vi "Pause Counter.vi"(8 "error in (no error)":errorcluster, 10 "ligne index":i32, 11 "Hardware Resources in":T1={"AI"={"task name"="", "task_ref"="", "physical channels"="Dev1/ai0:7", "channels config"={"input terminal configuration"=0, "minimum value"=-5.0, "maximum value"=5.0}, "rate"=1000.0}, "conversions"={"ai0"={"a"=0.0, "b"=0.0}, "ai1"={"a"=0.0, "b"=0.0}, "ai2"={"a"=0.0, "b"=0.0}, "ai3"={"a"=0.0, "b"=0.0}, "ai4"={"a"=0.0, "b"=0.0}}, "compteur 0"={"task name"="CTR", "task_ref"="", "ctr"="Dev1/ctr0:3", "coeff"=4000.0}, "compteur 1"={"task name"="CTR1", "task_ref"="", "ctr"="Dev1/ctr1", "coeff"=4000.0}, "compteur 2"={"task name"="CTR2", "task_ref"="", "ctr"="Dev1/ctr2", "coeff"=4000.0}, "compteur 3"={"task name"="CTR3", "task_ref"="", "ctr"="Dev1/ctr3", "coeff"=4000.0}} {"compteur 3"."coeff" format="%0.2f"; "compteur 2"."coeff" format="%0.2f"; "compteur 1"."coeff" format="%0.2f"; "compteur 0"."coeff" format="%0.2f"; "AI"."rate" format="%0.2f"; "AI"."channels config"."input terminal configuration" items=["Default"=-1, "RSE"=10083, "NRSE"=10078, "Differential"=10106, "Pseudodifferential"=12529]}) -> (0 "error out":errorcluster, 3 "Hardware Resources out":T1={"AI"={"task name"="", "task_ref"="", "physical channels"="Dev1/ai0:7", "channels config"={"input terminal configuration"=0, "minimum value"=-5.0, "maximum value"=5.0}, "rate"=1000.0}, "conversions"={"ai0"={"a"=0.0, "b"=0.0}, "ai1"={"a"=0.0, "b"=0.0}, "ai2"={"a"=0.0, "b"=0.0}, "ai3"={"a"=0.0, "b"=0.0}, "ai4"={"a"=0.0, "b"=0.0}}, "compteur 0"={"task name"="CTR", "task_ref"="", "ctr"="Dev1/ctr0:3", "coeff"=4000.0}, "compteur 1"={"task name"="CTR1", "task_ref"="", "ctr"="Dev1/ctr1", "coeff"=4000.0}, "compteur 2"={"task name"="CTR2", "task_ref"="", "ctr"="Dev1/ctr2", "coeff"=4000.0}, "compteur 3"={"task name"="CTR3", "task_ref"="", "ctr"="Dev1/ctr3", "coeff"=4000.0}} {"compteur 3"."coeff" format="%0.2f"; "compteur 2"."coeff" format="%0.2f"; "compteur 1"."coeff" format="%0.2f"; "compteur 0"."coeff" format="%0.2f"; "AI"."rate" format="%0.2f"; "AI"."channels config"."input terminal configuration" items=["Default"=-1, "RSE"=10083, "NRSE"=10078, "Differential"=10106, "Pseudodifferential"=12529]})   [LabVIEW 2014, in "PLS Acquisition.lvlib"]
doc: "Stops the acquisition."
uses:
  PLS Acquisition.lvlib
  Hardware Configuration.ctl
  Settings/conversion.ctl
  Settings/PLS Settings.lvlib
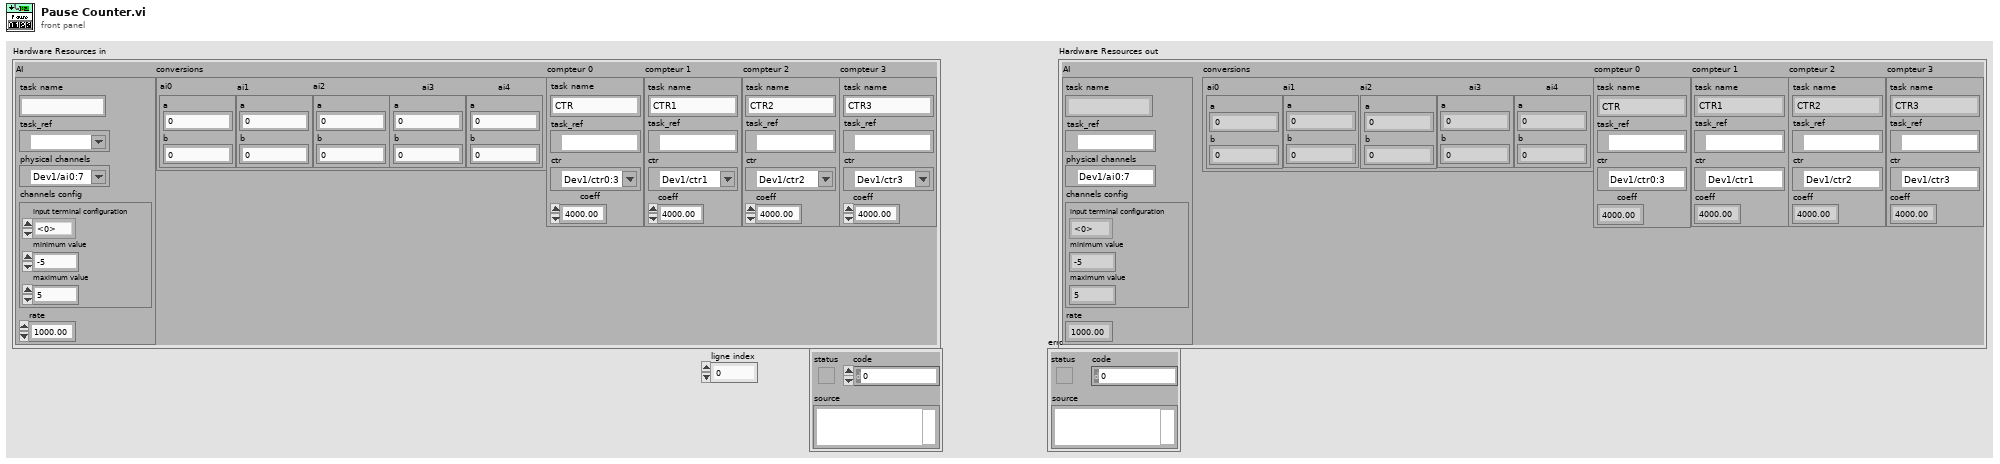
[diagram p1: front panel]
types:
  T1 = typedef "PLS Acquisition.lvlib/Hardware Configuration.ctl" = cluster{"AI":cluster{"task name":string, "task_ref":refnum<k21>, "physical channels":tag, "channels config":cluster{"input terminal configuration":i32, "minimum value":dbl, "maximum value":dbl}, "rate":dbl}, "conversions":cluster{"ai0":T2, "ai1":T2, "ai2":T2, "ai3":T2, "ai4":T2}, "compteur 0":cluster{"task name":string, "task_ref":refnum<k21>, "ctr":tag, "coeff":dbl}, "compteur 1":cluster{"task name":string, "task_ref":refnum<k21>, "ctr":tag, "coeff":dbl}, "compteur 2":cluster{"task name":string, "task_ref":refnum<k21>, "ctr":tag, "coeff":dbl}, "compteur 3":cluster{"task name":string, "task_ref":refnum<k21>, "ctr":tag, "coeff":dbl}}
  T2 = typedef "PLS Settings.lvlib/conversion.ctl" = cluster{"a":dbl, "b":dbl}
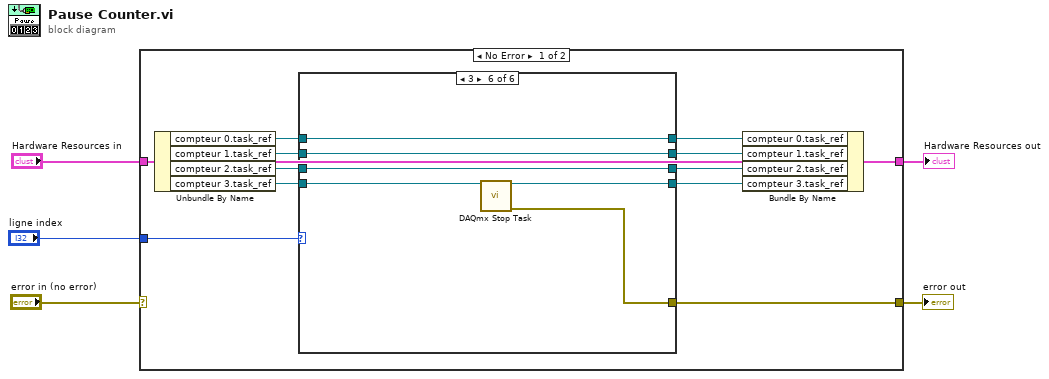
[diagram p0: block diagram]
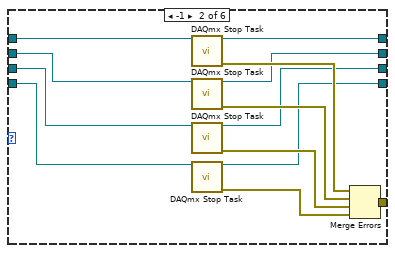
[diagram p3: hidden frame]
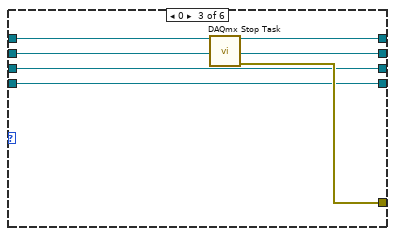
[diagram p4: hidden frame]
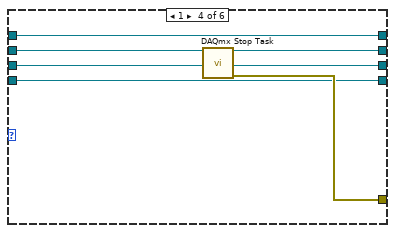
[diagram p5: hidden frame]
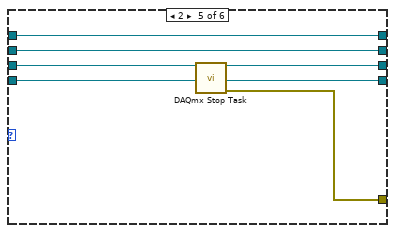
[diagram p6: hidden frame]
diagram:
  n1 = case shown="No Error" "error in (no error)" {
    selector: "error in (no error)" -> [_ w60]
    tunnel: [w17 w60] -> w4
    tunnel: "Hardware Resources in" -> [w11 w59]
    tunnel: "ligne index" -> [w12 _]
    tunnel: [w6 w59] -> w1
    frame No Error {
      n2 = Unbundle By Name(w11) -> ("compteur 0.task_ref"=w16:refnum<k21>, "compteur 1.task_ref"=w15:refnum<k21>, "compteur 2.task_ref"=w14:refnum<k21>, "compteur 3.task_ref"=w13:refnum<k21>)
      n3 = case shown="3" w12 {
        tunnel: [_ w34 w39 w45 w51 w57] -> w17
        tunnel: w16 -> [w21 w33 w40 w44 w50 w56]
        tunnel: w15 -> [w20 w31 w37 w46 w49 w55]
        tunnel: w14 -> [w19 w30 w36 w42 w52 w54]
        tunnel: w13 -> [w18 w27 w35 w41 w47 w58]
        tunnel: [w21 w25 w38 w44 w50 w56] -> w10
        tunnel: [w20 w24 w37 w43 w49 w55] -> w9
        tunnel: [w19 w23 w36 w42 w48 w54] -> w8
        tunnel: [w18 w22 w35 w41 w47 w53] -> w7
        frame Default {
        }
        frame -1 {
          n4 = call <vilib>:"DAQmx Stop Task.vi"("task/channels in"=w33) -> ("task out"=w25:refnum<k21>, "error out"=w32:errorcluster)  [unwired: 13 in]
          n5 = call <vilib>:"DAQmx Stop Task.vi"("task/channels in"=w31) -> ("task out"=w24:refnum<k21>, "error out"=w28:errorcluster)  [unwired: 13 in]
          n6 = call <vilib>:"DAQmx Stop Task.vi"("task/channels in"=w30) -> ("task out"=w23:refnum<k21>, "error out"=w29:errorcluster)  [unwired: 13 in]
          n7 = call <vilib>:"DAQmx Stop Task.vi"("task/channels in"=w27) -> ("task out"=w22:refnum<k21>, "error out"=w26:errorcluster)  [unwired: 13 in]
          n8 = Merge Errors(w32, w28, w29, w26) -> (w34:errorcluster)
        }
        frame 0 {
          n9 = call <vilib>:"DAQmx Stop Task.vi"("task/channels in"=w40) -> ("task out"=w38:refnum<k21>, "error out"=w39:errorcluster)  [unwired: 13 in]
        }
        frame 1 {
          n10 = call <vilib>:"DAQmx Stop Task.vi"("task/channels in"=w46) -> ("task out"=w43:refnum<k21>, "error out"=w45:errorcluster)  [unwired: 13 in]
        }
        frame 2 {
          n11 = call <vilib>:"DAQmx Stop Task.vi"("task/channels in"=w52) -> ("task out"=w48:refnum<k21>, "error out"=w51:errorcluster)  [unwired: 13 in]
        }
        frame 3 {
          n12 = call <vilib>:"DAQmx Stop Task.vi"("task/channels in"=w58) -> ("task out"=w53:refnum<k21>, "error out"=w57:errorcluster)  [unwired: 13 in]
        }
      }
      n13 = Bundle By Name(cluster=w11, "compteur 0.task_ref"=w10, "compteur 1.task_ref"=w9, "compteur 2.task_ref"=w8, "compteur 3.task_ref"=w7) -> (w6:T1)
    }
    frame Error {
    }
  }
  "error out" <- w4
  "Hardware Resources out" <- w1
